vi "akcelerometr.vi"() -> ()   [LabVIEW 2014]
doc: "This example demonstrates how to read X, Y, and Z accelerations using the MMA8452 accelerometer."
uses:
  <vilib>/MakerHub/LINX/LMH-LINX.lvlib
  <vilib>/MakerHub/LINX/Public/Utilities/Open Local.vi
panel:
  out "kąt wykres":dbl(graph)
  out "kąt nachylenia":dbl
  in  "Stop Button":bool
  out "Waveform Chart":T1(graph)
  out "Loop Rate (Hz)":u32
  # "LIS3DH Accelerometer\n\nThis example demonstrates how to read three axis of acceleration from the LIS3DH (MMA8452Q) accelerometer"
  # "Analog Value"
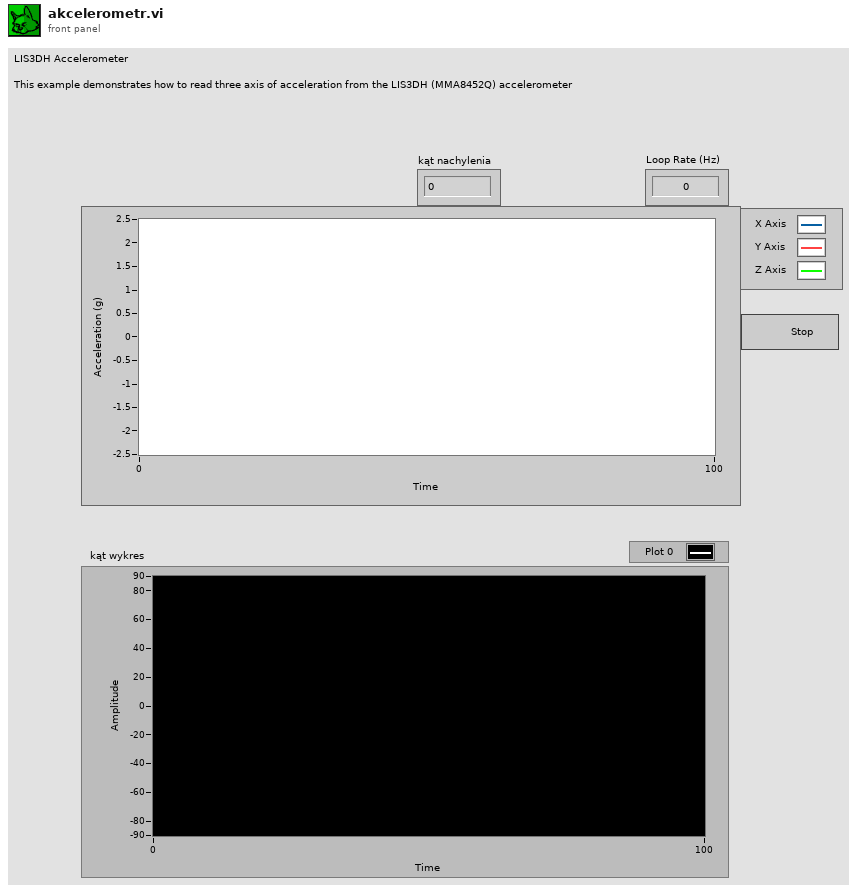
[diagram p1: front panel]
types:
  T1 = cluster{"X Axis":dbl, "Y Axis":dbl, "Z Axis":dbl}
  T2 = typedef "LMH-LINX.lvlib/LINX Ref.ctl" = cluster{"IO":T3, "Interface":T4, "LINX Device Config":T5}
  T3 = typedef "LMH-LINX.lvlib/Platform.ctl" = enum16{"Remote", "Local"}
  T4 = typedef "LMH-LINX.lvlib/Interface.ctl" = enum16{"Serial", "TCP"}
  T5 = typedef "LMH-LINX.lvlib/Device.lvlib/LINX Device Config.ctl" = cluster{"Interface":T4, "COM Port":refnum<visa-resource-name>, "TCP Configuration":T6, "Device Family":u8, "Device ID":u8, "Device Name":string, "TCP Ref":refnum<k5>, "Channels":T7}
  T6 = typedef "LMH-LINX.lvlib/Device.lvlib/TCP Config.ctl" = cluster{"IP Address":string, "Port":u16}
  T7 = typedef "LMH-LINX.lvlib/Channels.ctl" = cluster{"DI":u8[], "DO":u8[], "AI":u8[], "AO":u8[], "PWM":u8[], "QE":u8[], "UART":u8[], "I2C 2":u8[], "SPI":u8[], "CAN":u8[], "Servo":u8[], "AI Ref (V)":dbl, "AI Resolution (Bits)":u8, "AO Ref (V)":dbl, "AO Resolution (Bits)":u8}
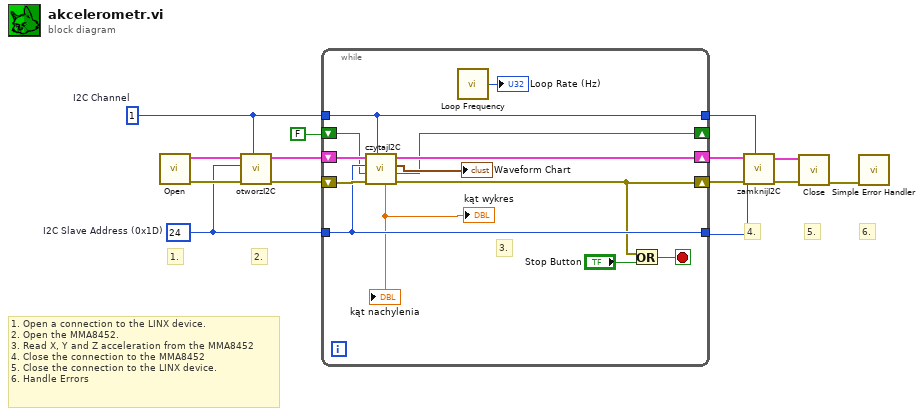
[diagram p0: block diagram]
diagram:
  w9 = u8 1  # I2C Channel
  w8 = u8 24  # I2C Slave Address (0x1D)
  # "6."
  # "4."
  # "2."
  # "5."
  # "1. Open a connection to the LINX device.\n2. Open the MMA8452.\n3. Read X, Y and Z acceleration from the MMA8452\n4. Close the connection to the MMA8452\n5. Close the connection to the LINX device.\n6. Handle Errors"
  # "1."
  n1 = call-poly <vilib>:"Open.vi"() -> ("Error Out"=w13:errorcluster, "LINX Resource"=w10:T2)  [unwired: 9 in, 1 out]
  n2 = call "otworzI2C.vi"("I2C Channel"=w9, "Error In"=w13, "I2C Slave Address (0x1D)"=w8, "LINX Ref"=w10) -> ("Error Out"=w12:errorcluster, "LINX Resource"=w11:T2)  [unwired: 6 in]
  n3 = while {
    tunnel: w9 -> [w21]
    tunnel: w8 -> [w23]
    shift-right: [w20] -> w2
    shift-left: w11 -> [w22]
    shift-right: [w19] -> w6
    shift-left: w12 -> [w24]
    tunnel: [w21] -> w3
    tunnel: [w23] -> w7
    shift-right: [w15] -> _
    shift-left: FALSE -> [w16]
    stop <- w26 stop-if-true
    # "3."
    n4 = call "czytajI2C.vi"("I2C Channel"=w21, "Error In"=w24, "Czy uśrednić?"=w16, "I2C Slave Address (0x1D)"=w23, "LINX Resource in"=w22) -> ("Error Out"=w19:errorcluster, "Czy kolejka pełna?"=w15:bool, "Acceleration Data (g)"=→"Waveform Chart":T1, "LINX Resource out"=w20:T2, "kąt nachylenia"=→"kąt nachylenia" →"kąt wykres":dbl)  [unwired: 2 in]
    n5 = call <vilib>:"Loop Frequency.vi"() -> ("Loop Rate (Hz)"=→"Loop Rate (Hz)":u32)
    n6 = Or(x=w19, y="Stop Button") -> (x .or. y?=w26:bool)
  }
  n7 = call "zamknijI2C.vi"("I2C Channel (0)"=w3, "Error In"=w6, "I2C Slave Address (0)"=w7, "LINX Resource"=w2) -> ("Error Out"=w5:errorcluster, "LINX Resource"=w4:T2)  [unwired: 6 in]
  n8 = call <vilib>:"Close.vi"("Error In"=w5, "LINX Resource"=w4) -> ("Error Out"=w14:errorcluster)  [unwired: 9 in]
  n9 = call <vilib>:"Simple Error Handler.vi"("error in (no error)"=w14) -> ()  [unwired: 4 in, 5 out]
